vi "Daily folder switch over process.vi"   [LabVIEW 2013]
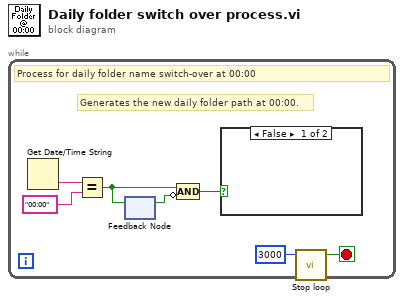
[diagram p0: block diagram]
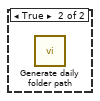
[diagram p2: hidden frame]
diagram:
  n1 = while {
    stop <- w7 stop-if-true
    # "Generates the new daily folder path at 00:00."
    # "Process for daily folder name switch-over at 00:00"
    n2 = Get Date/Time String() -> (time string=w4:string)  [unwired: 4 out]
    n3 = Equal?(x=w4, y="00:00" ("time string")) -> (x = y?=w3:bool)
    n4 = feedback-in #1(w3) -> ()
    n5 = feedback #1() -> (w2:bool)  [unwired: 1 in]
    n6 = Compound Arithmetic op=AND(w3, invert w2) -> (w1:bool)
    n7 = case shown="False" w1 {
      frame False {
      }
      frame True {
        n8 = call "Generate daily folder path.vi"() -> ()  [unwired: 11 in, 1 out]
      }
    }
    n9 = call "Stop loop.vi"("Loop iteration (ms)"=u32 3000) -> ("Stop"=w7:bool)  [unwired: 4 in]
  }
